vi "DontTip2.vi"(11 "Motor":cluster{"Right":dbl, "Left":dbl}) -> (2 "Left":dbl, 3 "Right":dbl)   [LabVIEW 2012]
uses:
  <vilib>/ptbypt/NI_PtbyPt.lvlib
panel:
  in  "Boolean":bool=TRUE
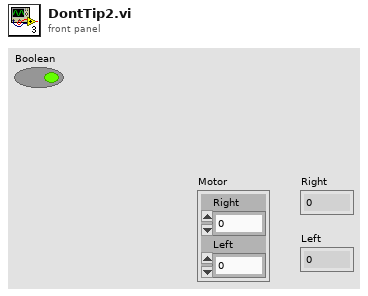
[diagram p1: front panel]
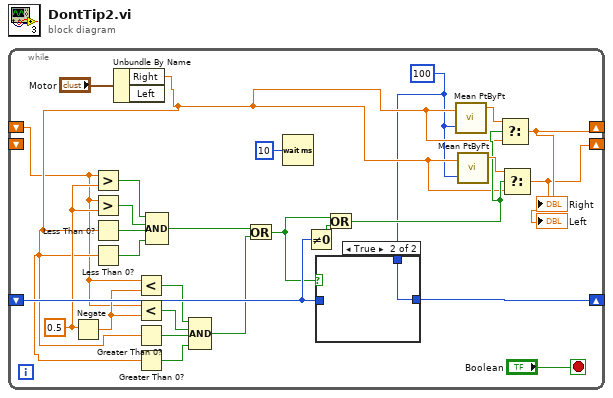
[diagram p0: block diagram]
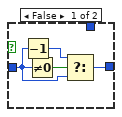
[diagram p2: hidden frame]
diagram:
  n1 = while {
    shift-right: [w20] -> _
    shift-left: _ -> [w2]
    shift-right: [w19] -> _
    shift-left: _ -> [_]
    shift-right: [w26] -> _
    shift-left: _ -> [w25]
    stop <- "Boolean" stop-if-true
    w6 = 0.5 ("y")
    w1 = 100 ("sample length")
    n2 = Negate(x=w6) -> (-x=w5:dbl)
    n3 = Greater?(x=w2, y=w6) -> (0:w18:bool)
    n4 = Greater?(x=w2, y=w6) -> (0:w17:bool)
    n5 = Unbundle By Name("Motor") -> ("Right"=w3:dbl)  [unwired: 1 out]
    n6 = Less Than 0?(x=w3) -> (x < 0?=w16:bool)
    n7 = Less Than 0?(x=w3) -> (x < 0?=w15:bool)
    n8 = Less?(x=w2, y=w5) -> (x < y?=w14:bool)
    n9 = Less?(x=w2, y=w5) -> (x < y?=w13:bool)
    n10 = Greater Than 0?(x=w3) -> (x > 0?=w12:bool)
    n11 = Greater Than 0?(x=w3) -> (x > 0?=w11:bool)
    n12 = Compound Arithmetic op=AND(w18, w17, w16, w15) -> (w10:bool)
    n13 = Compound Arithmetic op=AND(w14, w13, w12, w11) -> (w9:bool)
    n14 = Or(x=w10, y=w9) -> (x .or. y?=w4:bool)
    n15 = Wait (ms)(milliseconds to wait=u32 10) -> ()  [unwired: 1 out]
    n16 = Not Equal To 0?(x=w25) -> (x != 0?=w8:bool)
    n17 = case shown="True" w4 {
      tunnel: [w31 w32] -> w26
      tunnel: w25 -> [w28 _]
      tunnel: w1 -> [_ w32]
      frame False {
        n18 = Decrement(x=w28) -> (x-1=w29:i32)
        n19 = Not Equal To 0?(x=w28) -> (x != 0?=w30:bool)
        n20 = Select(t=w29, s=w30, f=w28) -> (s? t:f=w31:i32)
      }
      frame True {
      }
    }
    n21 = Or(x=w4, y=w8) -> (x .or. y?=w7:bool)
    n22 = call <vilib>:"Mean PtByPt.vi"("x"=w3, "sample length"=w1) -> ("mean"=w23:dbl)  [unwired: 2 in, 1 out]
    n23 = call <vilib>:"Mean PtByPt.vi"("x"=w3, "sample length"=w1) -> ("mean"=w24:dbl)  [unwired: 2 in, 1 out]
    n24 = Select(t=w23, s=w7, f=w3) -> (s? t:f=w20:dbl)
    "Right" <- w20
    n25 = Select(t=w24, s=w7, f=w3) -> (s? t:f=w19:dbl)
    "Left" <- w19
  }
